vi "Extract ROI Points.vi"(8 "error in (no error)":errorcluster, 10 "ROI Type":T1, 11 "String in":string) -> (0 "error out":errorcluster, 2 "Coordinates":i32[](array[numeric]), 3 "String out":string)   [LabVIEW 2021, in "Image.lvlib"]
uses:
  Image ROI Type.ctl
  Image.lvlib
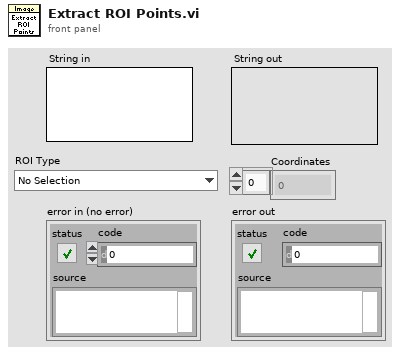
[diagram p1: front panel]
types:
  T1 = typedef "Image.lvlib/Image ROI Type.ctl" = enum16{"No Selection", "Point", "Line", "Rectangle", "Oval", "Polygon", "Freehand Region", "Annulus", "Unused2", "Unused3", "Broken Line", "Freehand Line", "Rotated Rectangle"}
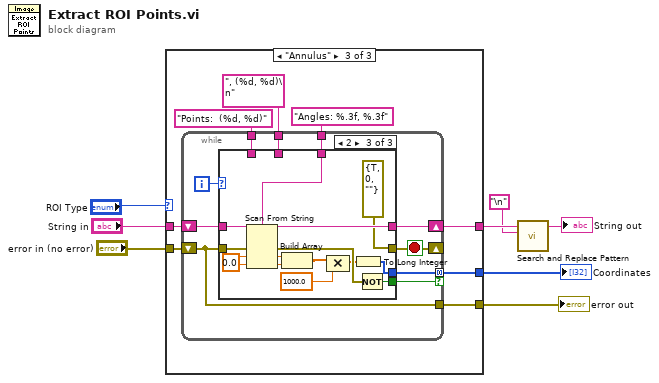
[diagram p0: block diagram]
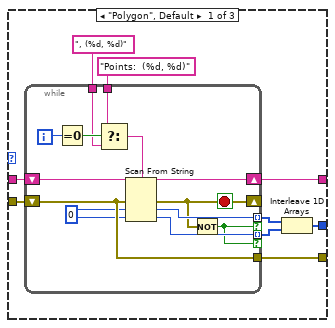
[diagram p2: hidden frame]
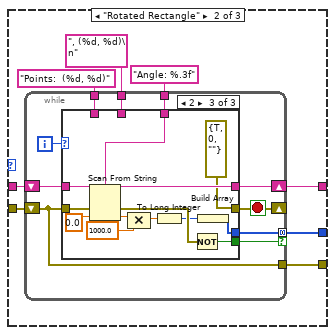
[diagram p3: hidden frame]
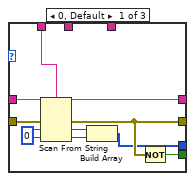
[diagram p4: hidden frame]
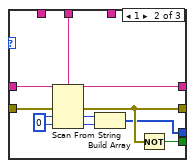
[diagram p5: hidden frame]
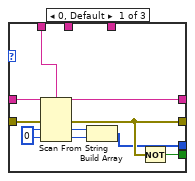
[diagram p6: hidden frame]
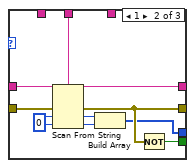
[diagram p7: hidden frame]
diagram:
  n1 = case shown="\"Annulus\"" "ROI Type" {
    tunnel: "String in" -> [w17 w38 w89]
    tunnel: "error in (no error)" -> [w16 w37 w88]
    tunnel: [w15 w36 w87] -> w6
    tunnel: [w12 w33 w84] -> w4
    tunnel: [w9 w32 w83] -> w1
    frame "Polygon", Default {
      n2 = while {
        shift-right: [w29] -> w12
        shift-left: w17 -> [w30]
        shift-right: [w18] -> _
        shift-left: w16 -> [w28]
        tunnel: [w28] -> w15
        tunnel: [w27] -> w11 mode=indexing if=w25
        tunnel: [w26] -> w10 mode=indexing if=w25
        tunnel: ", (%d, %d)" ("format string") -> [w22]
        tunnel: "Points:  (%d, %d)" ("format string") -> [w20]
        i -> [w24]
        stop <- w18 stop-if-true
        w19 = 0 ("Coordinates")
        n3 = Equal To 0?(x=w24) -> (x = 0?=w23:bool)
        n4 = Select(t=w20, s=w23, f=w22) -> (s? t:f=w21:string)
        n5 = Scan From String(format string=w21, input string=w30, error in=w28, default 1=w19, default 2=w19) -> (remaining string=w29:string, error out=w18:errorcluster, output 1=w27:i32, output 2=w26:i32)  [unwired: 1 in, 1 out]
        n6 = Not(x=w18) -> (.not. x?=w25:bool)
      }
      n7 = Interleave 1D Arrays(w11, w10) -> (w9:i32[])
    }
    frame "Rotated Rectangle" {
      n8 = while {
        shift-right: [w47] -> w33
        shift-left: w38 -> [w48]
        shift-right: [w41] -> _
        shift-left: w37 -> [w46]
        tunnel: [w46] -> w36
        tunnel: [w45] -> w32 mode=concatenating if=w44
        tunnel: ", (%d, %d)\n" ("format string") -> [w43]
        tunnel: "Points:  (%d, %d)" ("format string") -> [w42]
        tunnel: "Angle: %.3f" ("format string") -> [w39]
        i -> [w40]
        stop <- w41 stop-if-true
        n9 = case shown="2" w40 {
          tunnel: w48 -> [w58 w68 w81]
          tunnel: [w57 w67 w80] -> w47
          tunnel: w46 -> [w56 w66 w79]
          tunnel: [w49 w60 w74] -> w45
          tunnel: [w52 w62 w75] -> w44
          tunnel: w43 -> [_ w61 _]
          tunnel: w42 -> [w53 _ _]
          tunnel: [w54 w63 errorcluster {"status"=TRUE, "code"=0, "source"=""} ("error IO")] -> w41
          tunnel: w39 -> [_ _ w72]
          frame 0, Default {
            w55 = 0 ("Coordinates")
            n10 = Scan From String(format string=w53, input string=w58, error in=w56, default 1=w55, default 2=w55) -> (remaining string=w57:string, error out=w54:errorcluster, output 1=w51:i32, output 2=w50:i32)  [unwired: 1 in, 1 out]
            n11 = Build Array(w51, w50) -> (w49:i32[])
            n12 = Not(x=w54) -> (.not. x?=w52:bool)
          }
          frame 1 {
            w64 = 0 ("Coordinates")
            n13 = Scan From String(format string=w61, input string=w68, error in=w66, default 1=w64, default 2=w64) -> (remaining string=w67:string, error out=w63:errorcluster, output 1=w65:i32, output 2=w59:i32)  [unwired: 1 in, 1 out]
            n14 = Build Array(w65, w59) -> (w60:i32[])
            n15 = Not(x=w63) -> (.not. x?=w62:bool)
          }
          frame 2 {
            n16 = Scan From String(format string=w72, input string=w81, error in=w79, default 1=0.0 ("Coordinates")) -> (remaining string=w80:string, error out=w76:errorcluster, output 1=w78:dbl)  [unwired: 1 in, 1 out]
            n17 = Compound Arithmetic op=MULTIPLY(w78, 1000.0 ("value")) -> (w71:dbl)
            n18 = To Long Integer(number=w71) -> (32bit integer=w69:i32)
            n19 = Not(x=w76) -> (.not. x?=w75:bool)
            n20 = Build Array(w69) -> (w74:i32[])
          }
        }
      }
    }
    frame "Annulus" {
      n21 = while {
        shift-right: [w98] -> w84
        shift-left: w89 -> [w99]
        shift-right: [w92] -> _
        shift-left: w88 -> [w97]
        tunnel: [w97] -> w87
        tunnel: [w96] -> w83 mode=concatenating if=w95
        tunnel: ", (%d, %d)\n" ("format string") -> [w94]
        tunnel: "Points:  (%d, %d)" ("format string") -> [w93]
        tunnel: "Angles: %.3f, %.3f" ("format string") -> [w90]
        i -> [w91]
        stop <- w92 stop-if-true
        n22 = case shown="2" w91 {
          tunnel: w99 -> [w109 w119 w133]
          tunnel: [w108 w118 w132] -> w98
          tunnel: w97 -> [w107 w117 w131]
          tunnel: [w100 w111 w120] -> w96
          tunnel: [w103 w113 w129] -> w95
          tunnel: w94 -> [_ w112 _]
          tunnel: w93 -> [w104 _ _]
          tunnel: [w105 w114 errorcluster {"status"=TRUE, "code"=0, "source"=""} ("error IO")] -> w92
          tunnel: w90 -> [_ _ w127]
          frame 0, Default {
            w106 = 0 ("Coordinates")
            n23 = Scan From String(format string=w104, input string=w109, error in=w107, default 1=w106, default 2=w106) -> (remaining string=w108:string, error out=w105:errorcluster, output 1=w102:i32, output 2=w101:i32)  [unwired: 1 in, 1 out]
            n24 = Build Array(w102, w101) -> (w100:i32[])
            n25 = Not(x=w105) -> (.not. x?=w103:bool)
          }
          frame 1 {
            w115 = 0 ("Coordinates")
            n26 = Scan From String(format string=w112, input string=w119, error in=w117, default 1=w115, default 2=w115) -> (remaining string=w118:string, error out=w114:errorcluster, output 1=w116:i32, output 2=w110:i32)  [unwired: 1 in, 1 out]
            n27 = Build Array(w116, w110) -> (w111:i32[])
            n28 = Not(x=w114) -> (.not. x?=w113:bool)
          }
          frame 2 {
            w124 = 0.0 ("Coordinates")
            n29 = Scan From String(format string=w127, input string=w133, error in=w131, default 1=w124, default 2=w124) -> (remaining string=w132:string, error out=w130:errorcluster, output 1=w122:dbl, output 2=w123:dbl)  [unwired: 1 in, 1 out]
            n30 = Build Array(w122, w123) -> (w121:dbl[])
            n31 = Compound Arithmetic op=MULTIPLY(w121, 1000.0 ("value")) -> (w126:dbl[])
            n32 = To Long Integer(number=w126) -> (32bit integer=w120:i32[])
            n33 = Not(x=w130) -> (.not. x?=w129:bool)
          }
        }
      }
    }
  }
  "Coordinates" <- w1
  "error out" <- w6
  n34 = call <vilib>:"Search and Replace Pattern.vi"("string"=w4, "regular expression (\"\")"="\n") -> ("result string"=→"String out":string)  [unwired: 3 in, 1 out]
